vi "TimeInterpBoolean_New.vi"(11 "MaxTime":dbl=1.0) -> (3 "TimeInterpBoolean":T1)   [LabVIEW 2019, in "Trajectory_Library.lvlib"]
doc: "Create the data cluster for a TIME_INTERPOLATABLE_BOOLEAN.\n\nThe TimeInterpolatableBuffer provides an easy way to estimate past measurements. One application might be in conjunction with the DifferentialDrivePoseEstimator, where knowledge of the robot pose at the time when vision or other global measurement were recorded is necessary, or for recording the past angles of mechanisms as measured by encoders.\n\nThe TIME_INTERPOLATABLE_BOOLEAN stores and returns boolean values.\n\nInputs:\n - Max Time -- The maximum time (seconds) of data to store in the buffer.\n\nOutputs:\n - Time Inter Boolean -- Created data structure cluster"
uses:
  Trajectory_Library.lvlib
  TIME_INTERPOLATABLE_BOOLEAN.ctl
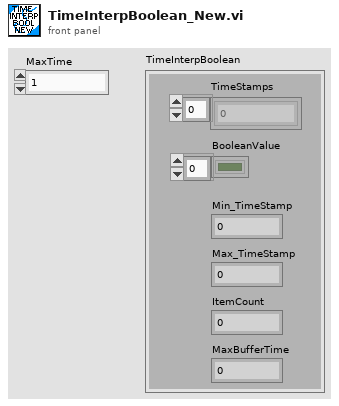
[diagram p1: front panel]
types:
  T1 = typedef "Trajectory_Library.lvlib/TIME_INTERPOLATABLE_BOOLEAN.ctl" = cluster{"TimeStamps":dbl[], "BooleanValue":bool[], "Min_TimeStamp":dbl, "Max_TimeStamp":dbl, "ItemCount":i32, "MaxBufferTime":dbl}
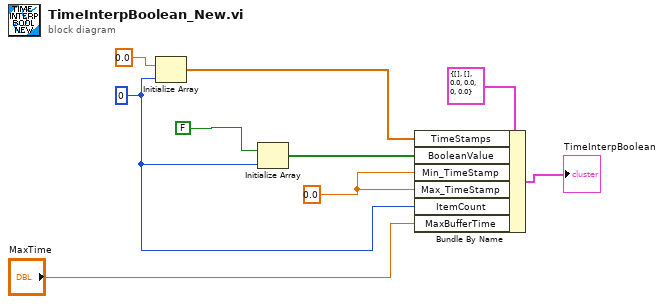
[diagram p0: block diagram]
diagram:
  w6 = 0.0 ("X")
  w3 = 0 ("dimension size")
  n1 = Initialize Array(0.0 ("element"), w3) -> (w7:dbl[])
  n2 = Initialize Array(FALSE, w3) -> (w4:bool[])
  n3 = Bundle By Name(cluster=T1 {"TimeStamps"=[], "BooleanValue"=[], "Min_TimeStamp"=0.0, "Max_TimeStamp"=0.0, "ItemCount"=0, "MaxBufferTime"=0.0} ("TIME_INTERPOLATABLE_DOUBLE"), "TimeStamps"=w7, "BooleanValue"=w4, "Min_TimeStamp"=w6, "Max_TimeStamp"=w6, "ItemCount"=w3, "MaxBufferTime"="MaxTime") -> (→"TimeInterpBoolean":T1)
